vi "E3A_Mov IDC.vi"(10 "Idc":dbl, 11 "SampleSize":i32=6) -> (3 "Mean":dbl format="%0.2f")   [LabVIEW 2022 SP3]
uses:
  <vilib>/Analysis/baseanly.llb/Mean (DBL).vi
  <vilib>/Analysis/NI_AALBase.lvlib
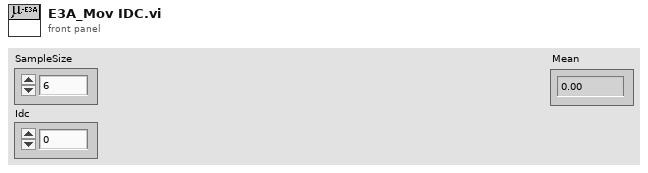
[diagram p1: front panel]
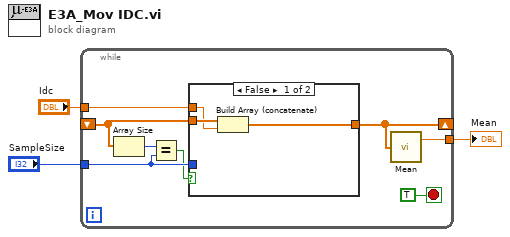
[diagram p0: block diagram]
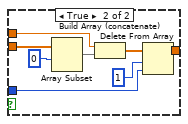
[diagram p2: hidden frame]
diagram:
  n1 = while {
    shift-right: [w5] -> _
    shift-left: _ -> [w11]
    tunnel: "SampleSize" -> [w9]
    tunnel: "Idc" -> [w8]
    tunnel: [w4] -> w1
    stop <- TRUE stop-if-true
    n2 = Array Size(array=w11) -> (size(s)=w10:i32)
    n3 = Equal?(x=w10, y=w9) -> (x = y?=w7:bool)
    n4 = case shown="False" w7 {
      tunnel: [w14 w18] -> w5
      tunnel: w11 -> [w13 w22]
      tunnel: w9 -> [_ w16]
      tunnel: w8 -> [w12 w15]
      frame False {
        n5 = Build Array (concatenate)(w13, w12) -> (w14:dbl[])
      }
      frame True {
        n6 = Array Subset(array=w22, index=0) -> (w20:dbl[])  [unwired: 1 in]
        n7 = Build Array (concatenate)(w15, w20) -> (w19:dbl[])
        n8 = Delete From Array(array=w19, length=1, index=w16) -> (array with subset deleted=w18:dbl[])  [unwired: 1 out]
      }
    }
    n9 = call-poly <vilib>:"Mean.vi"("X"=w5) -> ("mean"=w4:dbl)  [unwired: 1 out]
  }
  "Mean" <- w1
